vi "Calculate Equation.vi"() -> ()   [LabVIEW 2012]
panel:
  in  "C":dbl(knob) scale=0.0..10.0
  out "Gauge":dbl(knob) scale=0.0..200.0
  out "Meter":dbl(knob) scale=0.0..200.0
  in  "B":dbl(slide) scale=0.0..100.0
  in  "D":dbl(knob) scale=0.0..10.0
  in  "A":dbl(slide) scale=0.0..100.0
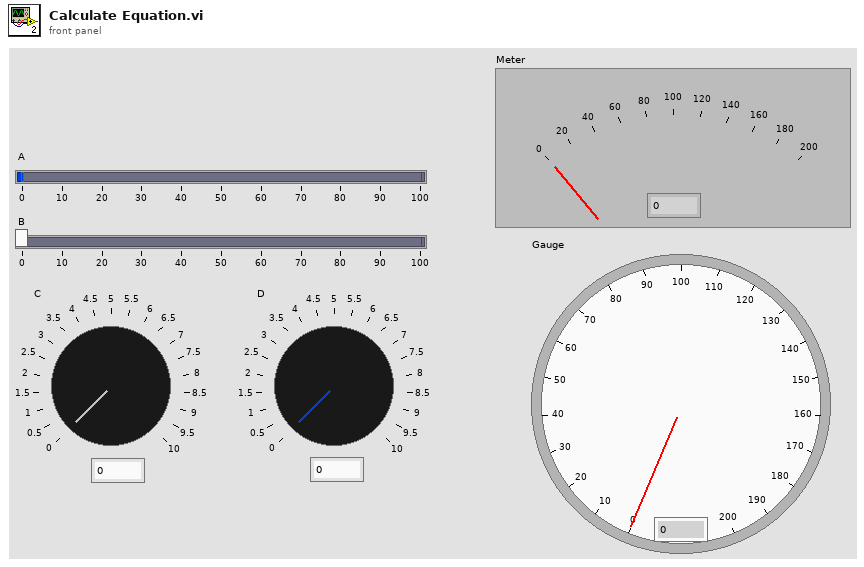
[diagram p1: front panel]
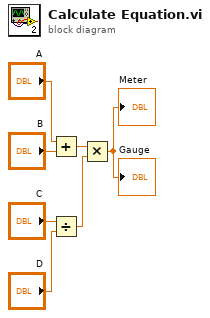
[diagram p0: block diagram]
diagram:
  n1 = Add(x="A", y="B") -> (x+y=w5:dbl)
  n2 = Divide(x="C", y="D") -> (x/y=w3:dbl)
  n3 = Multiply(x=w5, y=w3) -> (x*y=→"Meter" →"Gauge":dbl)
